vi "VariantToObject.vi"(8 "error in (no error)":errorcluster, 11 "Object":variant) -> (0 "error out":errorcluster, 1 "DecomposedObject":T1[](array[typedef]), 2 "Type":string, 3 "Value":string)   [LabVIEW 2019, in "BlueVariantView.lvlib"]
uses:
  BlueVariantView.lvlib
  DecomposedObject.ctl
  <vilib>/PNR/LabVIEW Composition/Composition/Composition.lvlib
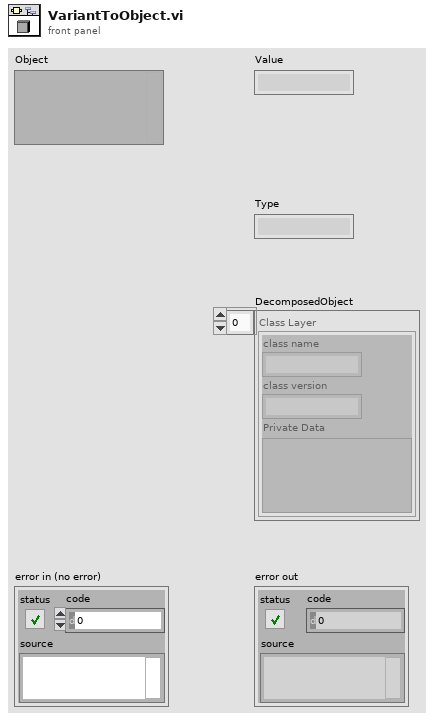
[diagram p1: front panel]
types:
  T1 = typedef "BlueVariantView.lvlib/DecomposedObject.ctl" = cluster{"class name":string, "class version":string, "Private Data":variant}
  T2 = cluster{"Major":u16, "Minor":u16, "Fix":u16, "Build":u16}[]
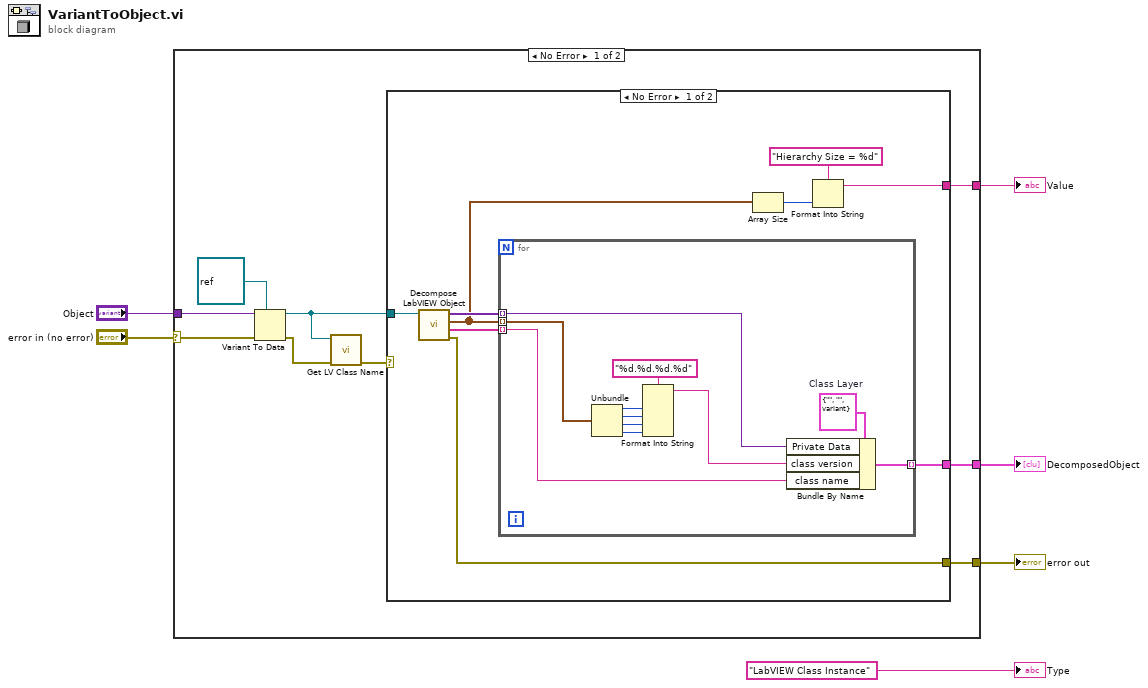
[diagram p0: block diagram]
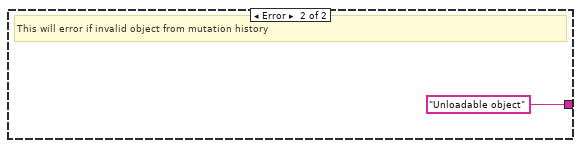
[diagram p2: hidden frame]
diagram:
  n1 = case shown="No Error" "error in (no error)" {
    selector: "error in (no error)" -> [w13 w37]
    tunnel: "Object" -> [w14 _]
    tunnel: [w12 _] -> w3
    tunnel: [w11 _] -> w2
    tunnel: [w10 w37] -> w1
    frame No Error {
      n2 = Variant To Data(error in=w13, type=refnum<class> refnum ("LabVIEW Object"), Variant=w14) -> (data=w8:refnum<class>, error out=w9:errorcluster)
      n3 = call <vilib>:"Get LV Class Name.vi"("error in (no error)"=w9, "object"=w8) -> ("error out"=w7:errorcluster)  [unwired: 8 in, 1 out]
      n4 = case shown="No Error" w7 {
        tunnel: [w19 _] -> w12
        tunnel: [w18 "Unloadable object"] -> w11
        tunnel: [w17 _] -> w10
        tunnel: w8 -> [w16 _]
        frame No Error {
          n5 = call <vilib>:"Decompose LabVIEW Object.vi"("LabVIEW Object"=w16) -> ("error out"=w17:errorcluster, "Class Names"=w20:string[], "Library Versions"=w21:T2, "Private Data Clusters"=w22:variant[])  [unwired: 7 in]
          n6 = for {
            tunnel: w22 -> [w34] mode=indexing
            tunnel: w21 -> [w30] mode=indexing
            tunnel: w20 -> [w33] mode=indexing
            tunnel: [w32] -> w19 mode=indexing
            w35 = T1 {"class name"="", "class version"="", "Private Data"=variant}  # Class Layer
            n7 = Unbundle(w30) -> ("Major"=w29:u16, "Minor"=w28:u16, "Fix"=w27:u16, "Build"=w26:u16)
            n8 = Format Into String(format string="%d.%d.%d.%d", w29, w28, w27, w26) -> (resulting string=w25:string)  [unwired: 2 in, 1 out]
            n9 = Bundle By Name(cluster=w35, "Private Data"=w34, "class version"=w25, "class name"=w33) -> (w32:T1)
          }
          n10 = Array Size(array=w21) -> (size(s)=w24:i32)
          n11 = Format Into String(format string="Hierarchy Size = %d", w24) -> (resulting string=w18:string)  [unwired: 2 in, 1 out]
        }
        frame Error {
          # "This will error if invalid object from mutation history"
        }
      }
    }
    frame Error {
    }
  }
  "error out" <- w1
  "Value" <- w2
  "DecomposedObject" <- w3
  "Type" <- "LabVIEW Class Instance" ("Type")
